vi "CS SQL Server.about me.vi"   [LabVIEW 2014, in "CS SQL Server.lvlib"]
doc: "VI used to display \"About me\" information."
uses:
  CS SQL Server.lvlib
  CSlibraries/UtilityLib/UtilityLib.helpType.ctl
  CSlibraries/UtilityLib/UtilityLib.lvlib
panel:
  # "Refer to block diagram!"
types:
  T1 = typedef "UtilityLib.lvlib/UtilityLib.helpType.ctl" = enum16{"unknown", "menu", "description", "about", "special0", "special1", "special2"}
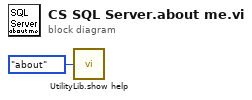
[diagram p0: block diagram]
diagram:
  n1 = call "UtilityLib.show help.vi"("helpType"=UtilityLib.helpType."about") -> ()
